vi "Cmd Execute.vi"(5 "cache size (1)":i32=1 min=1, 6 "error in (no error)":errorcluster, 7 "cursor type":T1, 9 "command reference":T3) -> (0 "error out":errorcluster, 3 "command-recordset reference":T2)   [LabVIEW 2013, in "NI_Database_API_64.lvlib"]
doc: "Executes an SQL query and returns a recordset reference that you must eventually free with the DB Tools Free Object VI. Wire data to the reference input to determine the polymorphic instance to use or manually select the instance."
uses:
  NI_Database_API_64.lvlib
  Cmd ObjectReference.ctl
  Command-Recordset.llb/Cmd-Rec Object Reference.ctl
  Auxilliary.llb/DB Tools Cursor Type.ctl
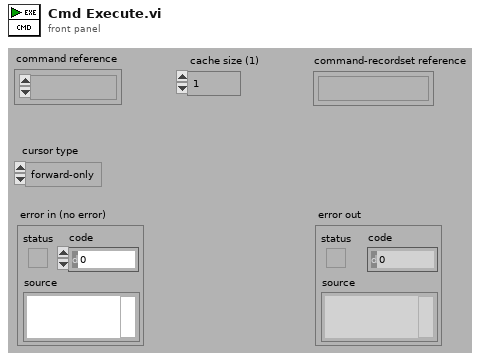
[diagram p1: front panel]
types:
  T1 = typedef "NI_Database_API_64.lvlib/DB Tools Cursor Type.ctl" = enum16{"forward-only", "keyset", "dynamic", "static"}
  T2 = typedef "NI_Database_API_64.lvlib/Cmd-Rec Object Reference.ctl" = refnum<k1>
  T3 = typedef "NI_Database_API_64.lvlib/Cmd ObjectReference.ctl" = refnum<k1>
  T4 = typedef "NI_Database_API_64.lvlib/Rec ObjectReference.ctl" = refnum<k1>
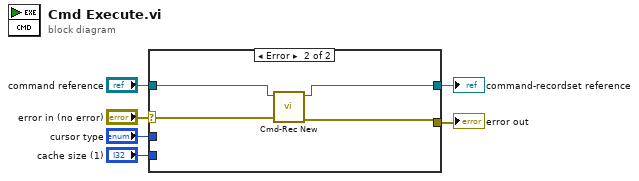
[diagram p0: block diagram]
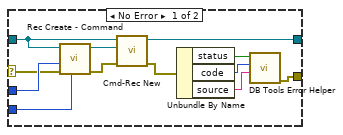
[diagram p2: hidden frame]
diagram:
  n1 = case shown="Error" "error in (no error)" {
    selector: "error in (no error)" -> [w7 w22]
    tunnel: "cursor type" -> [w18 _]
    tunnel: "cache size (1)" -> [w17 _]
    tunnel: "command reference" -> [w16 w19]
    tunnel: [w14 w20] -> w3
    tunnel: [w8 w21] -> w2
    frame No Error {
      n2 = call "Rec Create - Command.vi"("cache size (1)"=w17, "error in (no error)"=w7, "cursor type"=w18, "command reference"=w16) -> ("error out"=w13:errorcluster, "recordset reference"=w15:T4)  [unwired: 4 out]
      n3 = call "Cmd-Rec New.vi"("error in (no error)"=w13, "recordset reference"=w15, "command reference"=w16) -> ("error out"=w9:errorcluster, "command-recordset reference"=w14:T2)  [unwired: 3 out]
      n4 = Unbundle By Name(w9) -> ("status"=w11:bool, "code"=w10:i32, "source"=w12:string)
      n5 = call "DB Tools Error Helper.vi"("source"=w12, "code"=w10, "status"=w11) -> ("error out"=w8:errorcluster)  [unwired: 1 in, 7 out]
    }
    frame Error {
      n6 = call "Cmd-Rec New.vi"("error in (no error)"=w22, "command reference"=w19) -> ("error out"=w21:errorcluster, "command-recordset reference"=w20:T2)  [unwired: 1 in, 3 out]
    }
  }
  "error out" <- w2
  "command-recordset reference" <- w3
